vi "Find Custom Devices.vi"(8 "error in":errorcluster, 11 "target":refnum<k24>) -> (0 "error out":errorcluster, 2 "AIM ARINC 429 custom devices":T1[](array[typedef]) format="%.0x", 3 "target out":refnum<k24>)   [LabVIEW 2020, in "AIM ARINC 429 Scripting.lvlib"]
doc: "Within the specified target, this VI searches for all the AIM ARINC 429 custom devices and returns references to found <b>AIM ARINC 429 custom devices</b>."
uses:
  AIM ARINC 429 Scripting.lvlib
  NationalInstruments.VeriStand.SystemDefinitionAPI
  Constants.vi
  <vilib>/NI VeriStand/Custom Device API/Custom Device Item Ref.ctl
  <vilib>/NI VeriStand/Custom Device API/Custom Device API.lvlib
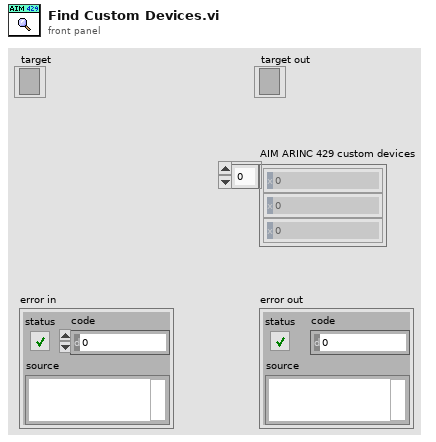
[diagram p1: front panel]
types:
  T1 = typedef "Custom Device API.lvlib/Custom Device Item Ref.ctl" = u64
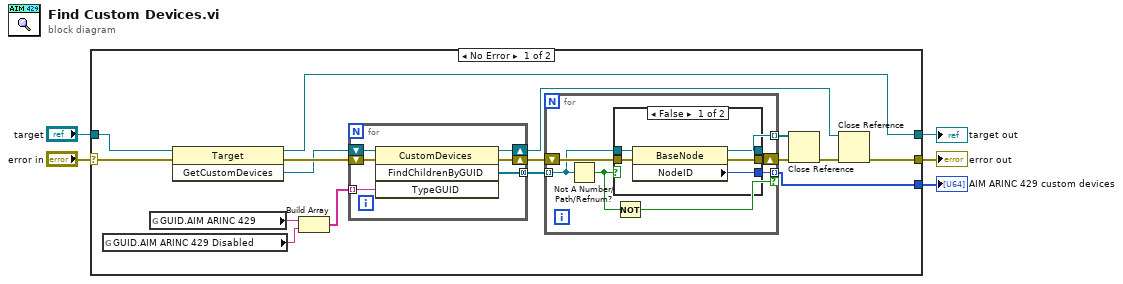
[diagram p0: block diagram]
diagram:
  n1 = case shown="No Error" "error in" {
    selector: "error in" -> [w15 w43]
    tunnel: "target" -> [w17 w42]
    tunnel: [w10 w43] -> w3
    tunnel: [w9 _] -> w1
    tunnel: [w12 w42] -> w2
    frame No Error {
      n2 = global read "Constants.vi" "GUID.AIM ARINC 429 Disabled"() -> (w7:string)
      n3 = global read "Constants.vi" "GUID.AIM ARINC 429"() -> (w8:string)
      n4 = invoke on="Invoke Node" class="Target" method="GetCustomDevices"(reference=w17, error in=w15) -> (reference out=w12:refnum<k24>, error out=w21:errorcluster, "GetCustomDevices"=w20:refnum<k24>)  [unwired: 1 in]
      n5 = Build Array(w8, w7) -> (w6:string[])
      n6 = for {
        tunnel: [w25] -> w16 mode=concatenating
        shift-right: [w23] -> w11
        shift-left: w21 -> [w27]
        shift-right: [w24] -> w13
        shift-left: w20 -> [w26]
        tunnel: w6 -> [w22] mode=indexing
        n7 = invoke on="Invoke Node" class="CustomDevices" method="FindChildrenByGUID"(reference=w26, error in=w27, "TypeGUID"=w22) -> (reference out=w24:refnum<k24>, error out=w23:errorcluster, "FindChildrenByGUID"=w25:refnum<k24>[])  [unwired: 1 in, 1 out]
      }
      n8 = for {
        shift-right: [w32] -> w18
        shift-left: w11 -> [w34]
        tunnel: w16 -> [w31] mode=indexing
        tunnel: [w33] -> w19 mode=indexing
        tunnel: [w30] -> w9 mode=indexing if=w28
        n9 = Not A Number/Path/Refnum?(number/path/refnum=w31) -> (NaN/Path/Refnum?=w29:bool)
        n10 = case shown="False" w29 {
          tunnel: [w36 w41] -> w32
          tunnel: w34 -> [w38 w41]
          tunnel: w31 -> [w39 w40]
          tunnel: [w37 w40] -> w33
          tunnel: [w35 _] -> w30
          frame False {
            n11 = property on="Property Node" class="BaseNode"(reference=w39, error in=w38) -> (reference out=w37:refnum<k24>, error out=w36:errorcluster, "NodeID"=w35:u64)
          }
          frame True {
          }
        }
        n12 = Not(x=w29) -> (.not. x?=w28:bool)
      }
      n13 = Close Reference(reference=w19, error in (no error)=w18) -> (error out=w14:errorcluster)
      n14 = Close Reference(reference=w13, error in (no error)=w14) -> (error out=w10:errorcluster)
    }
    frame Error {
    }
  }
  "error out" <- w3
  "target out" <- w2
  "AIM ARINC 429 custom devices" <- w1
